vi "SocketHook.vi"(0 "Socket_000 in":refnum<class "TCPAlerts.lvclass">, 2 "Mode":T1(ring), 7 "data in":string, 11 "error in (no error)":errorcluster) -> (4 "Socket_000 out":refnum<class "TCPAlerts.lvclass">, 8 "data out":string, 15 "error out":errorcluster)   [LabVIEW 2011, in "TCPAlerts.lvclass"]
uses:
  TCPAlerts.lvclass
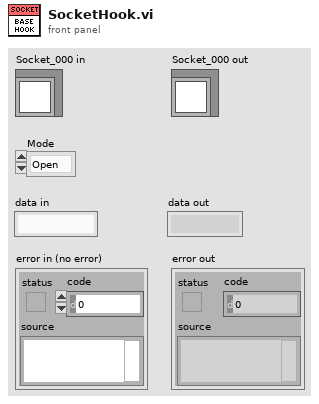
[diagram p1: front panel]
types:
  T1 = enum16{"Open", "R", "W", "R->W", "W->R", "Close"}
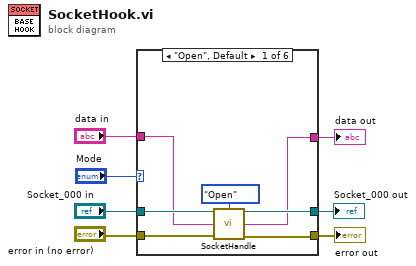
[diagram p0: block diagram]
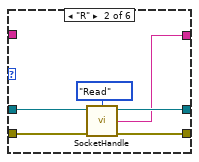
[diagram p2: hidden frame]
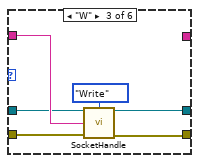
[diagram p3: hidden frame]
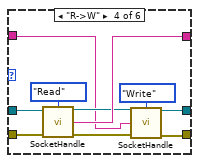
[diagram p4: hidden frame]
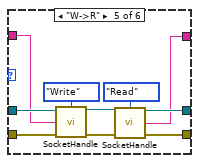
[diagram p5: hidden frame]
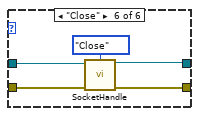
[diagram p6: hidden frame]
diagram:
  n1 = case shown="\"Open\", Default" "Mode" {
    tunnel: "error in (no error)" -> [w13 w18 w21 w34 w41 w48]
    tunnel: [w12 w19 w22 w27 w39 w47] -> w4
    tunnel: [w8 w15 _ w33 w37 _] -> w2
    tunnel: "data in" -> [w9 _ w25 w29 w38 _]
    tunnel: "Socket_000 in" -> [w11 w16 w24 w35 w42 w50]
    tunnel: [w10 w17 w23 w31 w40 w49] -> w5
    frame "Open", Default {
      n2 = call-dynamic "SocketHandle.vi"("Socket in"=w11, "Mode"=enum16{"Open", "Read", "Write", "Close"}."Open", "data in"=w9, "error in (no error)"=w13) -> ("Socket out"=w10:refnum<class "TCPAlerts.lvclass">, "data out"=w8:string, "error out"=w12:errorcluster)  [unwired: 9 in]
    }
    frame "R" {
      n3 = call-dynamic "SocketHandle.vi"("Socket in"=w16, "Mode"=enum16{"Open", "Read", "Write", "Close"}."Read", "error in (no error)"=w18) -> ("Socket out"=w17:refnum<class "TCPAlerts.lvclass">, "data out"=w15:string, "error out"=w19:errorcluster)  [unwired: 10 in]
    }
    frame "W" {
      n4 = call-dynamic "SocketHandle.vi"("Socket in"=w24, "Mode"=enum16{"Open", "Read", "Write", "Close"}."Write", "data in"=w25, "error in (no error)"=w21) -> ("Socket out"=w23:refnum<class "TCPAlerts.lvclass">, "error out"=w22:errorcluster)  [unwired: 9 in, 1 out]
    }
    frame "R->W" {
      n5 = call-dynamic "SocketHandle.vi"("Socket in"=w35, "Mode"=enum16{"Open", "Read", "Write", "Close"}."Read", "error in (no error)"=w34) -> ("Socket out"=w30:refnum<class "TCPAlerts.lvclass">, "data out"=w33:string, "error out"=w28:errorcluster)  [unwired: 10 in]
      n6 = call-dynamic "SocketHandle.vi"("Socket in"=w30, "Mode"=enum16{"Open", "Read", "Write", "Close"}."Write", "data in"=w29, "error in (no error)"=w28) -> ("Socket out"=w31:refnum<class "TCPAlerts.lvclass">, "error out"=w27:errorcluster)  [unwired: 9 in, 1 out]
    }
    frame "W->R" {
      n7 = call-dynamic "SocketHandle.vi"("Socket in"=w42, "Mode"=enum16{"Open", "Read", "Write", "Close"}."Write", "data in"=w38, "error in (no error)"=w41) -> ("Socket out"=w44:refnum<class "TCPAlerts.lvclass">, "error out"=w43:errorcluster)  [unwired: 9 in, 1 out]
      n8 = call-dynamic "SocketHandle.vi"("Socket in"=w44, "Mode"=enum16{"Open", "Read", "Write", "Close"}."Read", "error in (no error)"=w43) -> ("Socket out"=w40:refnum<class "TCPAlerts.lvclass">, "data out"=w37:string, "error out"=w39:errorcluster)  [unwired: 10 in]
    }
    frame "Close" {
      n9 = call-dynamic "SocketHandle.vi"("Socket in"=w50, "Mode"=enum16{"Open", "Read", "Write", "Close"}."Close", "error in (no error)"=w48) -> ("Socket out"=w49:refnum<class "TCPAlerts.lvclass">, "error out"=w47:errorcluster)  [unwired: 10 in, 1 out]
    }
  }
  "error out" <- w4
  "Socket_000 out" <- w5
  "data out" <- w2
